vi "Get configuration chain.vi"(8 "error in (no error)":errorcluster, 11 "waveform_FPGABase in":refnum<class "waveform_FPGA.lvclass">) -> (0 "error out":errorcluster, 1 "class name":string[](array[string]), 2 "configuration chain":variant[](array[variant]), 3 "waveform_FPGABase out":refnum<class "waveform_FPGA.lvclass">)   [LabVIEW 2012, in "waveform_FPGA.lvclass"]
doc: "Returns an array of variants containing the configuration clusters of each class in the inheritance chain (lowest child class first), together with an array of all class names in the inheritance chain.\n\nFor classes without configuration cluster, the configuration chain contains empty variants."
uses:
  waveform_FPGA.lvclass
  <vilib>/Distrio/Murmex/Murmex/Murmex.lvclass
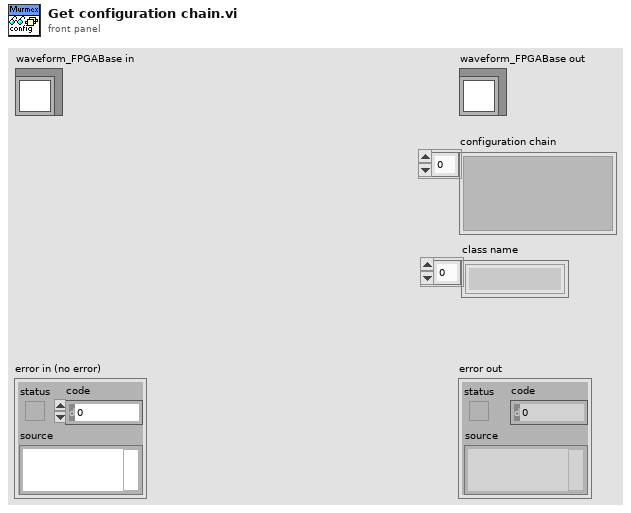
[diagram p1: front panel]
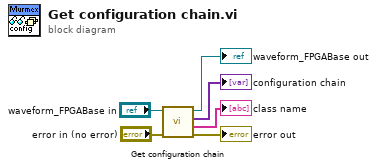
[diagram p0: block diagram]
diagram:
  n1 = call-parent "Get configuration chain.vi"("error in (no error)"="error in (no error)", "MurmexBase in"="waveform_FPGABase in") -> ("error out"=→"error out":errorcluster, "class name"=→"class name":string[], "configuration chain"=→"configuration chain":variant[], "MurmexBase out"=→"waveform_FPGABase out":refnum<class "waveform_FPGA.lvclass">)  [unwired: 6 in]
